vi "OutputControl.vi"(11 "输出控制":bool) -> ()   [LabVIEW 2020, in "YP03-60CurrentSource_1.lvlib"]
uses:
  YP03-60CurrentSource_1.lvlib
  <vilib>/Instr/_visa.llb/VISA Configure Serial Port (Instr).vi
panel:
  in  "error in (no error)":errorcluster
  out "String":string
  out "read buffer":string
  out "error out":errorcluster
  in  "Cluster":T1={"parity (0:none)"=enum."None", "data bits (8)"=8, "baud rate (9600)"=9600, "VISA resource name"="COM6"} {"data bits (8)" min=5 max=8 step=1}
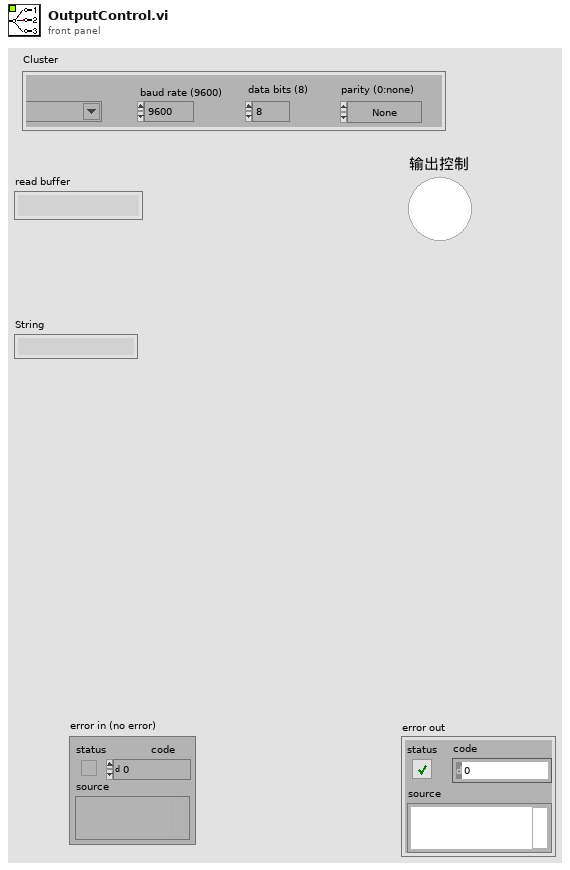
[diagram p1: front panel]
types:
  T1 = cluster{"parity (0:none)":enum16{"None", "Odd", "Even", "Mark", "Space"}, "data bits (8)":u16, "baud rate (9600)":u32, "VISA resource name":refnum<visa-resource-name>}
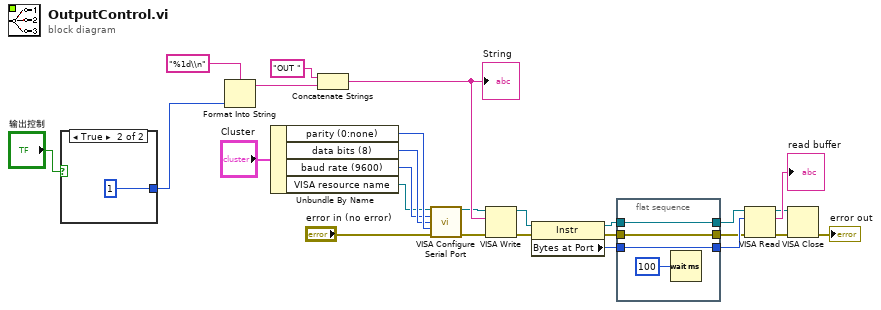
[diagram p0: block diagram]
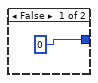
[diagram p2: hidden frame]
diagram:
  n1 = case shown="True" "输出控制" {
    tunnel: [0 1] -> w1
    frame False {
    }
    frame True {
    }
  }
  n2 = Format Into String(format string="%1d\\n", w1) -> (resulting string=w19:string)  [unwired: 2 in, 1 out]
  n3 = Unbundle By Name("Cluster") -> ("parity (0:none)"=w26:enum16{"None", "Odd", "Even", "Mark", "Space"}, "data bits (8)"=w25:u16, "baud rate (9600)"=w24:u32, "VISA resource name"=w23:refnum<visa-resource-name>)
  n4 = Concatenate Strings("OUT " ("string"), w19) -> (w15:string)
  "String" <- w15
  n5 = call-poly "VISA Configure Serial Port"("VISA resource name"=w23, "baud rate (9600)"=w24, "data bits (8)"=w25, "parity (0:none)"=w26, "error in (no error)"="error in (no error)") -> ("VISA resource name out"=w7:refnum<visa-resource-name>, "error out"=w6:errorcluster)  [unwired: 9 in]
  n6 = VISA Write(VISA resource name=w7, write buffer=w15, error in (no error)=w6) -> (VISA resource name out=w17:refnum<visa-resource-name>, error out=w16:errorcluster)  [unwired: 1 out]
  n7 = property class="Instr"(reference=w17, error in=w16) -> (reference out=w11:refnum<visa-resource-name>, error out=w9:errorcluster, "Bytes at Port"=w13:u32)
  n8 = flat-sequence {
    tunnel: w11 -> [w32]
    tunnel: [w32] -> w10
    tunnel: [w31] -> w8
    tunnel: w9 -> [w31]
    tunnel: [w30] -> w12
    tunnel: w13 -> [w30]
    frame #0 {
      n9 = Wait (ms)(milliseconds to wait=u32 100) -> ()  [unwired: 1 out]
    }
  }
  n10 = VISA Read(VISA resource name=w10, byte count=w12, error in (no error)=w8) -> (VISA resource name out=w3:refnum<visa-resource-name>, read buffer=→"read buffer":string, error out=w4:errorcluster)  [unwired: 1 out]
  n11 = VISA Close(VISA resource name=w3, error in (no error)=w4) -> (error out=→"error out":errorcluster)
